vi "Full adder.vi"() -> ()   [LabVIEW 2015]
panel:
  in  "input 3":bool
  out "S":bool
  in  "input 2":bool
  in  "input 1":bool
  out "C":bool
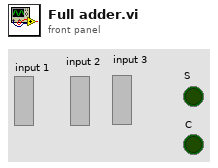
[diagram p1: front panel]
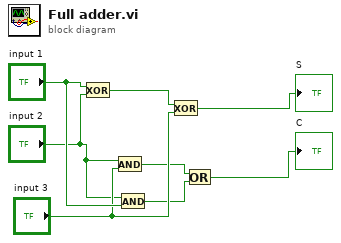
[diagram p0: block diagram]
diagram:
  n1 = Exclusive Or(1:"input 2", 2:"input 1") -> (0:w6:bool)
  n2 = And(x="input 2", y="input 3") -> (x .and. y?=w2:bool)
  n3 = And(x="input 2", y="input 1") -> (x .and. y?=w3:bool)
  n4 = Exclusive Or(1:"input 3", 2:w6) -> (0:→"S":bool)
  n5 = Or(x=w2, y=w3) -> (x .or. y?=→"C":bool)
